vi "Add E2E to configuration search paths.vi"(10 "Variant":variant) -> (0 "error out":errorcluster)   [LabVIEW 2015]
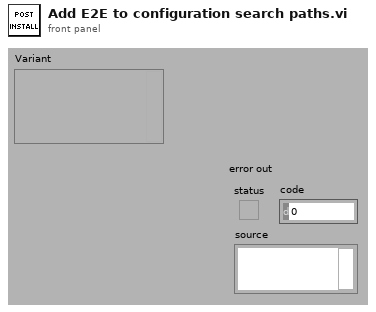
[diagram p1: front panel]
types:
  T1 = typedef "PL_class cache.lvlib/cache definition.ctl" = cluster{"configuration":T2, "class cache data":T3}
  T2 = typedef "PL_class cache.lvlib/cache search configuration.ctl" = cluster{"Search Paths":path[], "Folders to Exclude":string[], "full class list":path[]}
  T3 = typedef "PL_class cache.lvlib/cached class information.ctl" = cluster{"targets":T4[], "engines":T5[], "modules":T5[], "ignored class list":path[]}
  T4 = typedef "PL_class cache.lvlib/target class metadata.ctl" = cluster{"file name":string, "fully qualified name":string, "menu display name":string, "configuration class name":string}
  T5 = typedef "PL_class cache.lvlib/class metadata.ctl" = cluster{"file name":string, "fully qualified name":string, "menu display name":string, "configuration class":string, "category":string, "instances allowed":i32, "supported targets":T6[]}
  T6 = typedef "TBM configuration.lvclass/Target Types.ctl" = enum16{"Windows", "Mac", "Linux", "Linux RT ARM", "VxWorks", "Pharlap", "Other", "Linux RT x64"}
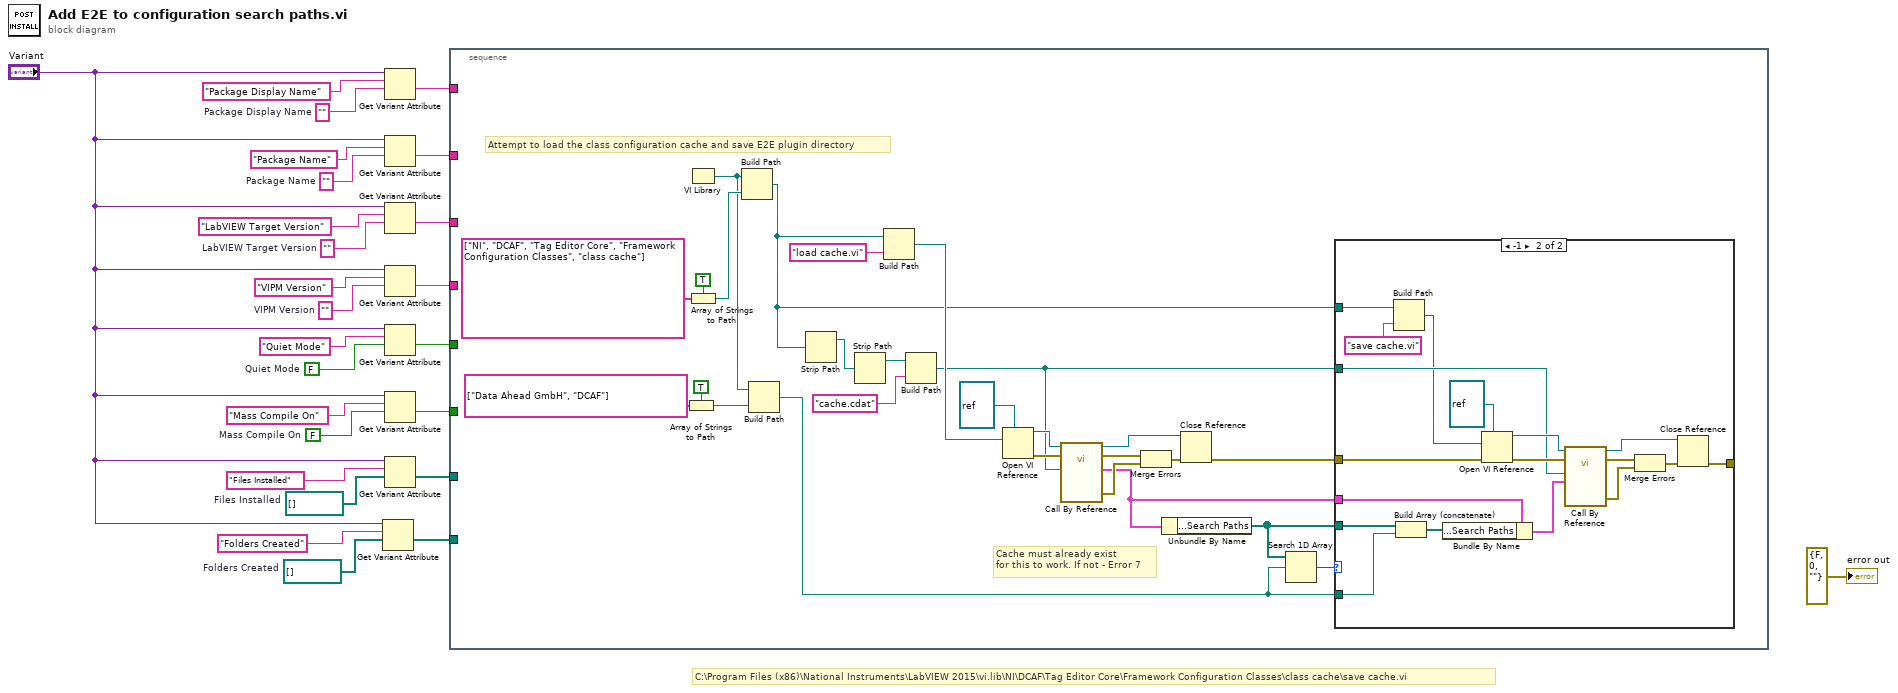
[diagram p0: block diagram]
diagram:
  w1 = path[] []  # Folders Created
  w2 = path[] []  # Files Installed
  w8 = FALSE  # Mass Compile On
  w9 = ""  # Package Display Name
  w16 = FALSE  # Quiet Mode
  w19 = ""  # VIPM Version
  w21 = ""  # LabVIEW Target Version
  w23 = ""  # Package Name
  # "C:\\Program Files (x86)\\National Instruments\\LabVIEW 2015\\vi.lib\\NI\\DCAF\\Tag Editor Core\\Framework Configuration Classes\\class cache\\save cache.vi"
  n1 = Get Variant Attribute(Variant="Variant", name="Folders Created", default value (empty Variant)=w1) -> (value=w6:path[])  [unwired: 1 in, 3 out]
  n2 = Get Variant Attribute(Variant="Variant", name="Package Display Name", default value (empty Variant)=w9) -> (value=w15:string)  [unwired: 1 in, 3 out]
  n3 = Get Variant Attribute(Variant="Variant", name="Package Name", default value (empty Variant)=w23) -> (value=w14:string)  [unwired: 1 in, 3 out]
  n4 = Get Variant Attribute(Variant="Variant", name="LabVIEW Target Version", default value (empty Variant)=w21) -> (value=w13:string)  [unwired: 1 in, 3 out]
  n5 = Get Variant Attribute(Variant="Variant", name="VIPM Version", default value (empty Variant)=w19) -> (value=w12:string)  [unwired: 1 in, 3 out]
  n6 = Get Variant Attribute(Variant="Variant", name="Quiet Mode", default value (empty Variant)=w16) -> (value=w11:bool)  [unwired: 1 in, 3 out]
  n7 = Get Variant Attribute(Variant="Variant", name="Mass Compile On", default value (empty Variant)=w8) -> (value=w10:bool)  [unwired: 1 in, 3 out]
  n8 = Get Variant Attribute(Variant="Variant", name="Files Installed", default value (empty Variant)=w2) -> (value=w5:path[])  [unwired: 1 in, 3 out]
  n9 = stacked-sequence {
    tunnel: w15 -> [_]
    tunnel: w14 -> [_]
    tunnel: w13 -> [_]
    tunnel: w12 -> [_]
    tunnel: w11 -> [_]
    tunnel: w10 -> [_]
    tunnel: w5 -> [_]
    tunnel: w6 -> [_]
    frame #0 {
      # "Cache must already exist\nfor this to work. If not - Error 7"
      # "Attempt to load the class configuration cache and save E2E plugin directory"
      n10 = Array of Strings to Path(0:string[] ["Data Ahead GmbH", "DCAF"], 1:TRUE ("relative")) -> (2:w29:path)
      n11 = VI Library() -> (path=w27:path)
      n12 = Array of Strings to Path(0:string[] ["NI", "DCAF", "Tag Editor Core", "Framework Configuration Classes", "class cache"], 1:TRUE ("relative")) -> (2:w50:path)
      n13 = Build Path(base path=w27, name or relative path=w50) -> (appended path=w32:path)
      n14 = Build Path(base path=w27, name or relative path=w29) -> (appended path=w28:path)
      n15 = Strip Path(path=w32) -> (stripped path=w44:path)  [unwired: 1 out]
      n16 = Strip Path(path=w44) -> (stripped path=w43:path)  [unwired: 1 out]
      n17 = Build Path(base path=w32, name or relative path="load cache.vi") -> (appended path=w47:path)
      n18 = Build Path(base path=w43, name or relative path="cache.cdat") -> (appended path=w33:path)
      n19 = Open VI Reference(type specifier VI Refnum (for type only)=refnum<vi> refnum, vi path=w47) -> (vi reference=w45:refnum<vi>, error out=w46:errorcluster)  [unwired: 4 in]
      n20 = call-by-ref "?"(reference=w45, error in=w46, "cache path"=w33) -> (reference out=w38:refnum<vi>, error out=w41:errorcluster, 0:"error out"=w40:errorcluster, "cache"=w35:T1)  [unwired: 9 in]
      n21 = Merge Errors(w41, w40) -> (w39:errorcluster)
      n22 = Unbundle By Name(w35) -> ("configuration.Search Paths"=w36:path[])
      n23 = Close Reference(reference=w38, error in (no error)=w39) -> (error out=w34:errorcluster)
      n24 = Search 1D Array(1D array=w36, element=w28) -> (index of element=w37:i32)  [unwired: 1 in]
      n25 = case shown="-1" w37 {
        tunnel: w36 -> [_ w71]
        tunnel: w35 -> [_ w69]
        tunnel: w34 -> [w53 w67]
        tunnel: w33 -> [_ w63]
        tunnel: w32 -> [_ w61]
        tunnel: w28 -> [_ w55]
        tunnel: [w53 w54] -> _
        frame Default {
        }
        frame -1 {
          n26 = Build Path(base path=w61, name or relative path="save cache.vi") -> (appended path=w60:path)
          n27 = Build Array (concatenate)(w71, w55) -> (w70:path[])
          n28 = Bundle By Name(cluster=w69, "configuration.Search Paths"=w70) -> (w64:T1)
          n29 = Open VI Reference(type specifier VI Refnum (for type only)=refnum<vi> refnum, vi path=w60, error in (no error)=w67) -> (vi reference=w65:refnum<vi>, error out=w66:errorcluster)  [unwired: 3 in]
          n30 = call-by-ref "?"(reference=w65, error in=w66, "cache"=w64, "path"=w63) -> (reference out=w56:refnum<vi>, error out=w59:errorcluster, 0:"error out"=w58:errorcluster)  [unwired: 9 in]
          n31 = Merge Errors(w59, w58) -> (w57:errorcluster)
          n32 = Close Reference(reference=w56, error in (no error)=w57) -> (error out=w54:errorcluster)
        }
      }
    }
  }
  "error out" <- errorcluster {"status"=FALSE, "code"=0, "source"=""} ("error out")
